vi "提示栏.vi"(0 "Enable":bool=TRUE caption="启用", 5 "error in (no error)":errorcluster caption="错误输入（无错误）") -> (13 "是否创建报表":bool, 14 "湿度下限":dbl format="%#g", 15 "湿度上限":dbl format="%#g", 16 "温度下限":dbl format="%#g", 17 "温度上限":dbl format="%#g", 18 "输入":bool, 19 "error out":errorcluster caption="错误输出")   [LabVIEW 2014]
doc: "显示标准对话框，提示用户输入用户名、密码等信息。\n--------------------\n\n该Express VI配置如下:\n\n显示给用户的信息:请输入“温度上限” “温度下限” “湿度上限” “湿度下限” 当温度湿度超出范围是会触发报警。\n该输入为: \n数字: 温度上限\n数字: 温度下限\n数字: 湿度上限\n数字: 湿度下限\n复选框: 是否创建报表"
panel:
  in  "是否创建报表":bool
  in  "湿度下限":u8(slide) scale=0.0..100.0
  in  "湿度上限":u8(slide)=100 scale=0.0..100.0
  in  "温度下限":u8(slide) scale=0.0..100.0
  in  "温度上限":u8(slide)=100 scale=0.0..100.0
  out "String":string="请输入“温度上限” “温度下限” “湿度上限” “湿度下限” 当温度湿度超出范围是会触发报警。" caption="字符串"
  in  "Cancel":bool caption="取消"
  in  "OK2":bool
  in  "OK1":bool
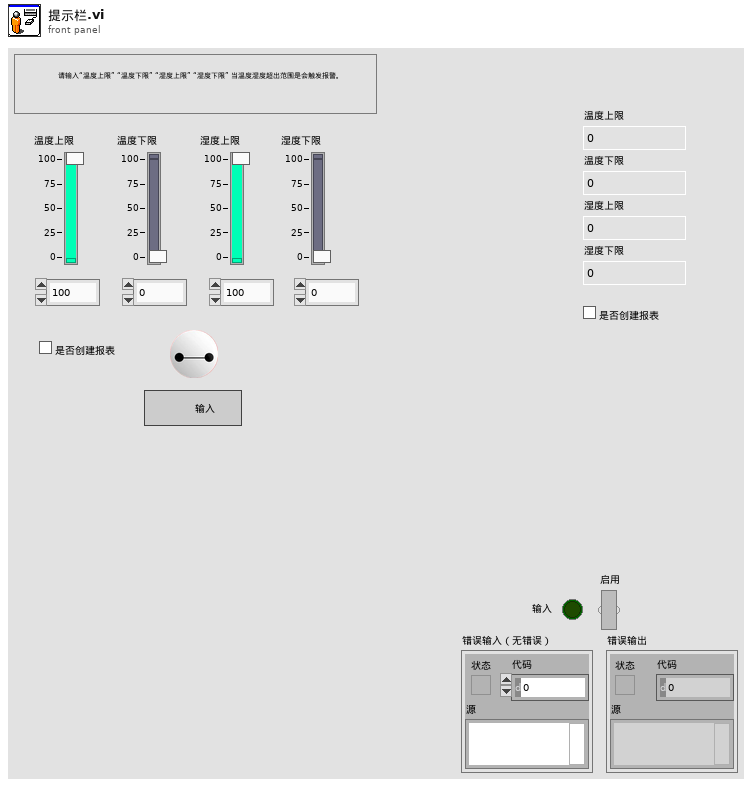
[diagram p1: front panel]
types:
  T1 = cluster{"Input Name":string, "Input Data Type":i32}[]
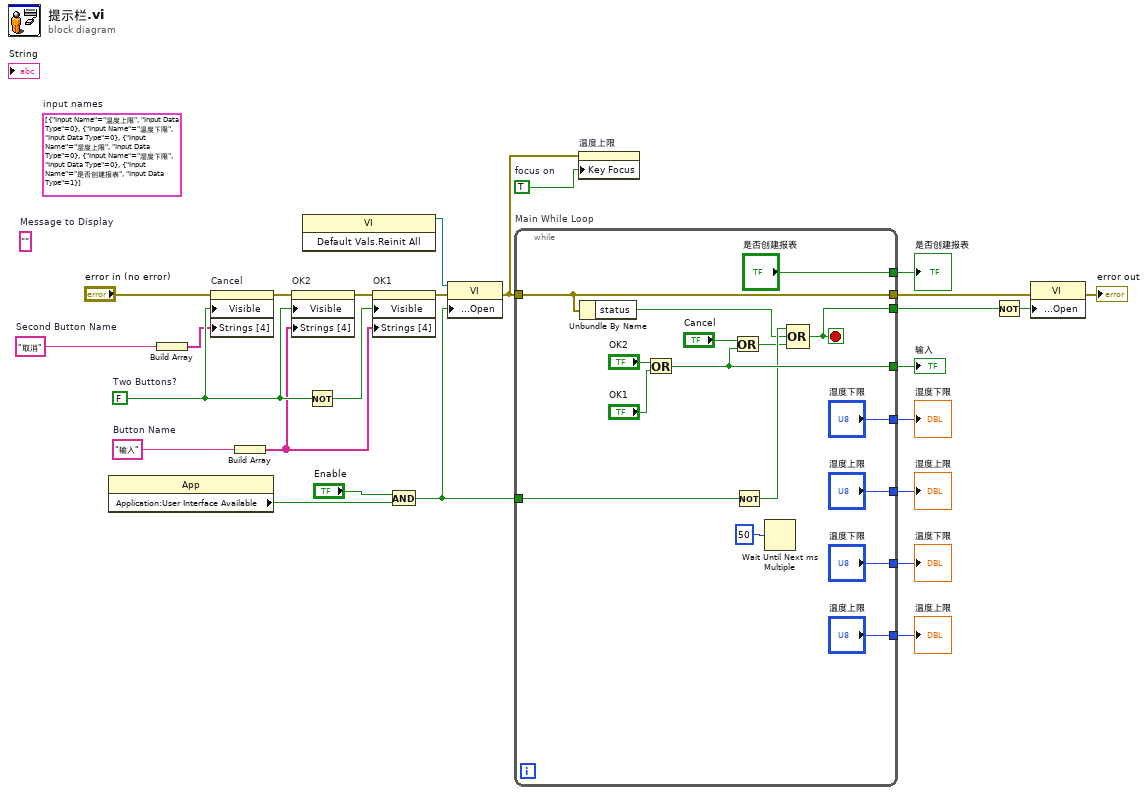
[diagram p0: block diagram]
diagram:
  w5 = TRUE  # focus on
  (unwired) T1 [{"Input Name"="温度上限", "Input Data Type"=0}, {"Input Name"="温度下限", "Input Data Type"=0}, {"Input Name"="湿度上限", "Input Data Type"=0}, {"Input Name"="湿度下限", "Input Data Type"=0}, {"Input Name"="是否创建报表", "Input Data Type"=1}]  # input names
  w18 = "取消"  # Second Button Name
  w16 = "输入"  # Button Name
  (unwired) ""  # Message to Display
  w26 = FALSE  # Two Buttons?
  n1 = property class="App"() -> ("Application:User Interface Available"=w8:bool)  [unwired: 2 in, 2 out]
  n2 = Build Array(w18) -> (w19:string[])
  n3 = property on="Cancel" class="Bool"(error in="error in (no error)", "Visible"=w26, "Strings [4]"=w19) -> (error out=w23:errorcluster)  [unwired: 1 in, 1 out]
  n4 = Build Array(w16) -> (w17:string[])
  n5 = property on="OK2" class="Bool"(error in=w23, "Visible"=w26, "Strings [4]"=w17) -> (error out=w22:errorcluster)  [unwired: 1 in, 1 out]
  n6 = invoke class="VI" method="Default Vals.Reinit All"() -> (reference out=w7:refnum<vi>)  [unwired: 3 in, 2 out]
  n7 = Not(x=w26) -> (.not. x?=w24:bool)
  n8 = property on="OK1" class="Bool"(error in=w22, "Visible"=w24, "Strings [4]"=w17) -> (error out=w15:errorcluster)  [unwired: 1 in, 1 out]
  n9 = And(x="Enable", y=w8) -> (x .and. y?=w9:bool)
  n10 = property class="VI"(reference=w7, error in=w15, "Front Panel Window:Open"=w9) -> (error out=w14:errorcluster)  [unwired: 1 out]
  n11 = while "Main While Loop" {
    tunnel: [w39] -> w25
    tunnel: w9 -> [w37]
    tunnel: [w35] -> w20
    tunnel: w14 -> [w34]
    tunnel: [w34] -> w12
    tunnel: ["温度上限"] -> w6
    tunnel: ["温度下限"] -> w4
    tunnel: ["湿度上限"] -> w3
    tunnel: ["湿度下限"] -> w2
    tunnel: ["是否创建报表"] -> w1
    stop <- w35 stop-if-true
    n12 = Unbundle By Name(w34) -> ("status"=w32:bool)
    n13 = Or(x="OK2", y="OK1") -> (x .or. y?=w39:bool)
    n14 = Or(x="Cancel", y=w39) -> (x .or. y?=w33:bool)
    n15 = Not(x=w37) -> (.not. x?=w36:bool)
    n16 = Wait Until Next ms Multiple(millisecond multiple=u32 50) -> ()  [unwired: 1 out]
    n17 = Compound Arithmetic op=OR(w36, w32, w33) -> (w35:bool)
  }
  "输入" <- w25
  "温度上限" <- w6
  "温度下限" <- w4
  "湿度上限" <- w3
  "湿度下限" <- w2
  "是否创建报表" <- w1
  n18 = property on="温度上限" class="Slide (严格)"(error in=w14, "Key Focus"=w5) -> ()  [unwired: 1 in, 2 out]
  n19 = Not(x=w20) -> (.not. x?=w21:bool)
  n20 = property class="VI"(error in=w12, "Front Panel Window:Open"=w21) -> (error out=→"error out":errorcluster)  [unwired: 1 in, 1 out]
